vi "FindAllMethods.vi"(8 "error in (no error)":errorcluster, 11 "CS++Actor in":refnum<class "CS++Actor.lvclass">) -> (0 "error out":errorcluster, 3 "CS++Actor out":refnum<class "CS++Actor.lvclass">)   [LabVIEW 2014, in "CS++Actor.lvlib" / "CS++Actor.lvclass"]
doc: "Searches for all public VIs in the actor."
uses:
  CS++Actor.lvclass
  CS++Actor.lvclass/CS++Actor.ctl
  CSPP_Method/CS++Method.lvclass
  CSPP_Method/CS++Method.lvclass/CS++Method.ctl
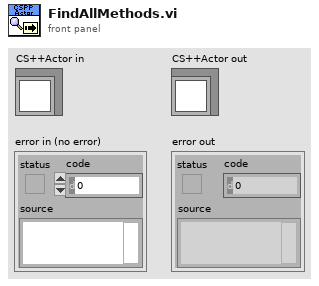
[diagram p1: front panel]
types:
  T1 = enum32{"invalid VI type", "Standard VI", "Control VI", "Global VI", "Polymorphic VI", "Configuration VI", "SubSystem", "Facade VI", "Method VI", "Statechart Diagram VI"}
  T2 = enum32{"invalid scope", "public", "private", "protected", "community"}
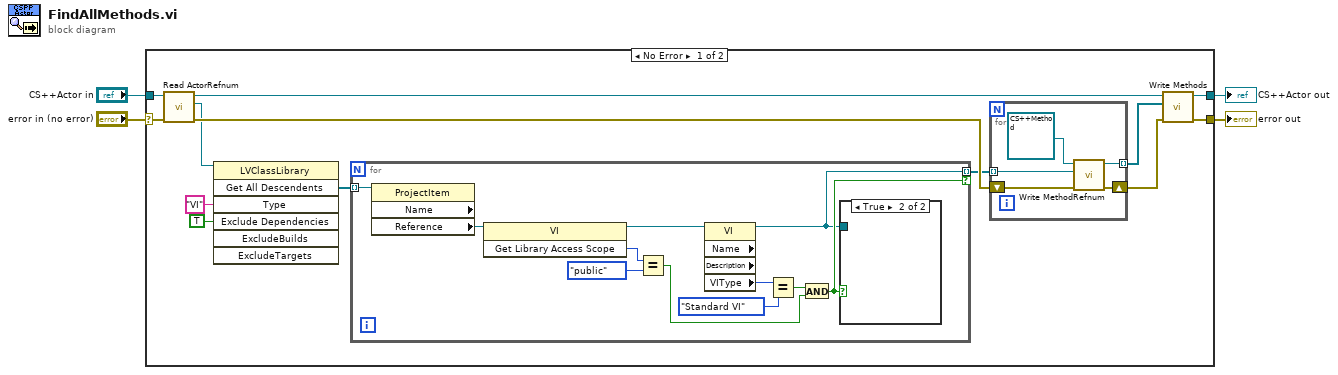
[diagram p0: block diagram]
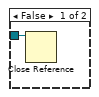
[diagram p2: hidden frame]
diagram:
  n1 = case shown="No Error" "error in (no error)" {
    selector: "error in (no error)" -> [w13 w36]
    tunnel: [w10 w36] -> w3
    tunnel: [w8 w35] -> w1
    tunnel: "CS++Actor in" -> [w14 w35]
    frame No Error {
      n2 = call "Read ActorRefnum.vi"("error in (no error)"=w13, "CS++Actor in"=w14) -> ("error out"=w11:errorcluster, "ActorRefnum"=w6:refnum<vi>, "CS++Actor out"=w9:refnum<class "CS++Actor.lvclass">)  [unwired: 7 in]
      n3 = invoke class="LVClassLibrary" method="Get All Descendents"(reference=w6, "Type"="VI", "Exclude Dependencies"=TRUE ("ExcludeDependencies")) -> ("All Descendents"=w15:refnum<vi>[])  [unwired: 4 in, 6 out]
      n4 = for {
        tunnel: w15 -> [w32] mode=indexing
        tunnel: [w23] -> w5 mode=indexing if=w24
        n5 = property class="ProjectItem" props=["Name", "Reference"](reference=w32) -> ("Reference"=w33:refnum<vi>)  [unwired: 1 in, 3 out]
        n6 = invoke class="VI" method="Get Library Access Scope"(reference=w33) -> (reference out=w26:refnum<vi>, "Get Library Access Scope"=w30:T2)  [unwired: 2 in, 1 out]
        n7 = Equal?(x=w30, y=T2."public") -> (x = y?=w25:bool)
        n8 = property class="VI" props=["Name", "Description", "VIType"](reference=w26) -> (reference out=w23:refnum<vi>, "VIType"=w29:T1)  [unwired: 1 in, 3 out]
        n9 = Equal?(x=w29, y=T1."Standard VI") -> (x = y?=w28:bool)
        n10 = And(x=w28, y=w25) -> (x .and. y?=w24:bool)
        n11 = case shown="True" w24 {
          tunnel: w23 -> [w34 _]
          frame False {
            n12 = Close Reference(reference=w34) -> ()  [unwired: 1 in, 1 out]
          }
          frame True {
          }
        }
      }
      n13 = for {
        shift-right: [w22] -> w12
        shift-left: w11 -> [w21]
        tunnel: [w19] -> w7 mode=indexing
        tunnel: w5 -> [w18] mode=indexing
        n14 = call "Write MethodRefnum.vi"("error in (no error)"=w21, "MethodRefnum"=w18, "CS++Methods in"=refnum<class "CS++Method.lvclass"> refnum ("CS++Method.lvlib:CS++Method.lvclass")) -> ("error out"=w22:errorcluster, "CS++Methods out"=w19:refnum<class "CS++Method.lvclass">)  [unwired: 7 in]
      }
      n15 = call "Write Methods.vi"("error in (no error)"=w12, "Methods"=w7, "CS++Actor in"=w9) -> ("error out"=w10:errorcluster, "CS++Actor out"=w8:refnum<class "CS++Actor.lvclass">)  [unwired: 7 in]
    }
    frame Error {
    }
  }
  "error out" <- w3
  "CS++Actor out" <- w1
